vi "Configure Electrical Calibration.vi"(5 "Unknown Thru (F: Disabled)":bool, 7 "Channel (1)":i32=1, 8 "error in (no error)":errorcluster, 9 "Characterization (0: Char 0)":u16(ring) items=["Char 0", "Char 1", "Char 2", "Char 3", "Char 4", "Char 5"], 10 "Isolating Measurement (F: Disabled)":bool, 11 "VISA resource name":refnum<visa-resource-name>) -> (0 "error out":errorcluster, 3 "VISA resource name out":refnum<visa-resource-name>)   [LabVIEW 2022 SP3, in "Agilent ENA Series.lvlib"]
doc: "Configures the electrical calibration."
uses:
  <instrlib>/Agilent ENA Series/Agilent ENA Series.lvlib
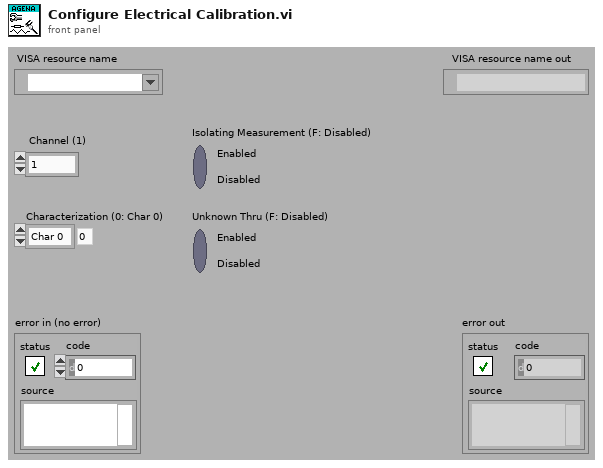
[diagram p1: front panel]
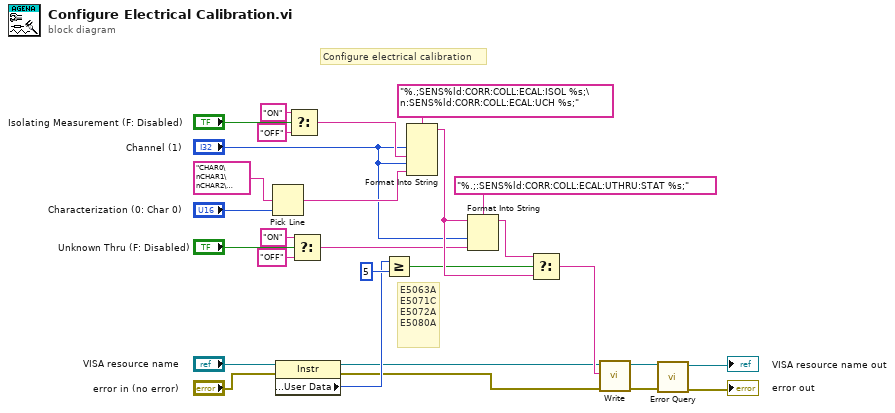
[diagram p0: block diagram]
diagram:
  # "E5063A\nE5071C\nE5072A\nE5080A"
  # "Configure electrical calibration"
  n1 = Pick Line(multi-line string="CHAR0\nCHAR1\nCHAR2\nCHAR3\nCHAR4\nCHAR5", line index="Characterization (0: Char 0)") -> (output string=w21:string)  [unwired: 1 in]
  n2 = property class="Instr"(reference="VISA resource name", error in="error in (no error)") -> (reference out=w2:refnum<visa-resource-name>, error out=w1:errorcluster, "General Settings:User Data"=w4:u32)
  n3 = Select(t="ON", s="Isolating Measurement (F: Disabled)", f="OFF") -> (s? t:f=w24:string)
  n4 = Select(t="ON", s="Unknown Thru (F: Disabled)", f="OFF") -> (s? t:f=w8:string)
  n5 = Greater Or Equal?(x=w4, y=u32 5) -> (x >= y?=w3:bool)
  n6 = Format Into String(format string="%.;SENS%ld:CORR:COLL:ECAL:ISOL %s;\n:SENS%ld:CORR:COLL:ECAL:UCH %s;", "Channel (1)", w24, "Channel (1)", w21) -> (resulting string=w12:string)  [unwired: 2 in, 1 out]
  n7 = Format Into String(format string="%.;:SENS%ld:CORR:COLL:ECAL:UTHRU:STAT %s;", initial string=w12, "Channel (1)", w8) -> (resulting string=w13:string)  [unwired: 1 in, 1 out]
  n8 = Select(t=w13, s=w3, f=w12) -> (s? t:f=w11:string)
  n9 = call <instrlib>:"Write.vi"("error in (no error)"=w1, "String ()"=w11, "VISA resource name"=w2) -> ("error out"=w19:errorcluster, "VISA resource name out"=w20:refnum<visa-resource-name>)  [unwired: 6 in, 1 out]
  n10 = call <instrlib>:"Error Query.vi"("error in (no error)"=w19, "VISA resource name"=w20) -> ("error out"=→"error out":errorcluster, "VISA resource name out"=→"VISA resource name out":refnum<visa-resource-name>)  [unwired: 6 in, 2 out]
